vi "Readexecution_count.vi"(8 "error in (no error)":errorcluster, 11 "object in":refnum<class "execute_input Message.lvclass">) -> (0 "error out":errorcluster, 2 "execution_count":u32, 3 "object out":refnum<class "execute_input Message.lvclass">)   [LabVIEW 2018, in "ClientMessaging.lvlib" / "execute_input Message.lvclass"]
uses:
  execute_input Message.lvclass
  execute_input Message.lvclass/execute_input Message.ctl
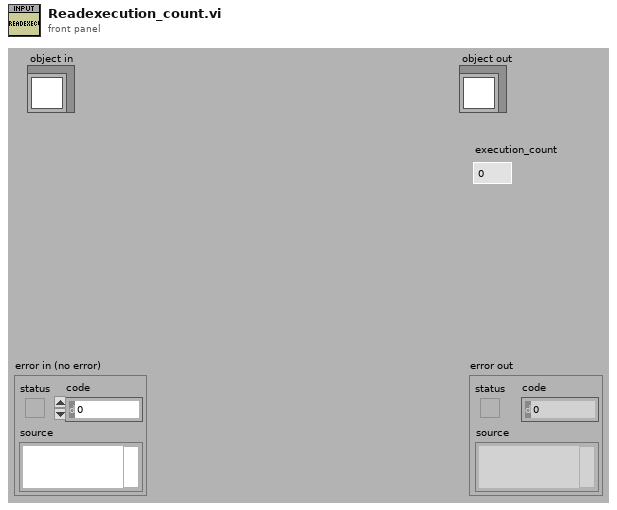
[diagram p1: front panel]
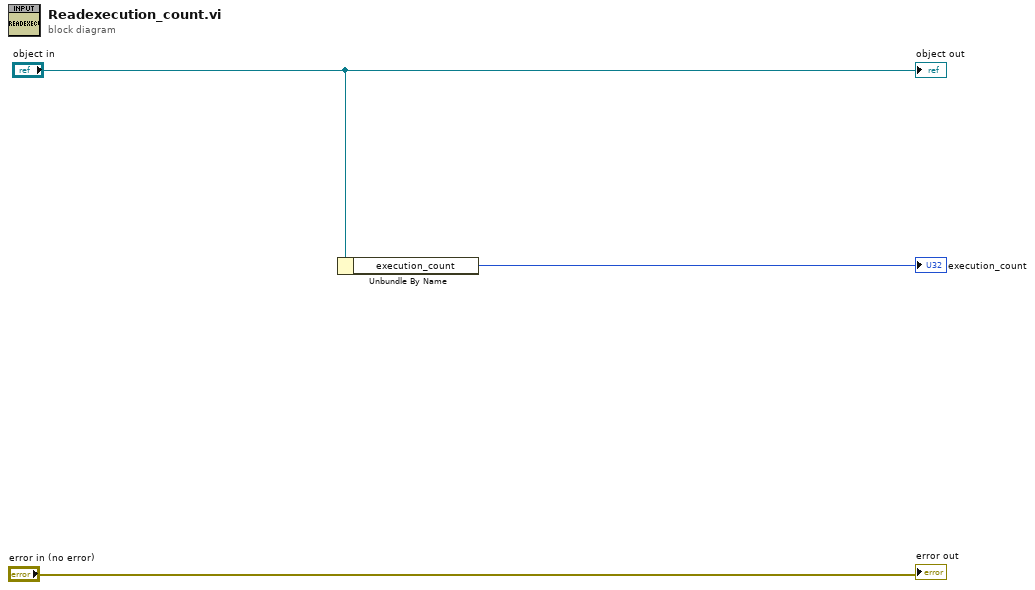
[diagram p0: block diagram]
diagram:
  n1 = Unbundle By Name("object in") -> ("execution_count"=→"execution_count":u32)
  "error out" <- "error in (no error)"
  "object out" <- "object in"
